vi "積分器(SubVI).vi"(6 "輸入累加ERR回朔":dbl, 7 "I增益":dbl=0.01, 9 "samples (Hz)":dbl, 10 "前一個ERR":dbl, 11 "當下ERR":dbl) -> (1 "輸出累加ERR回朔":dbl, 3 "積分修正量":dbl)   [LabVIEW 2010]
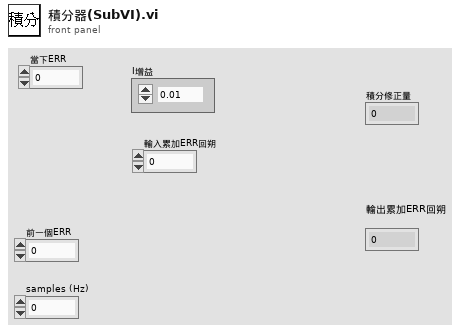
[diagram p1: front panel]
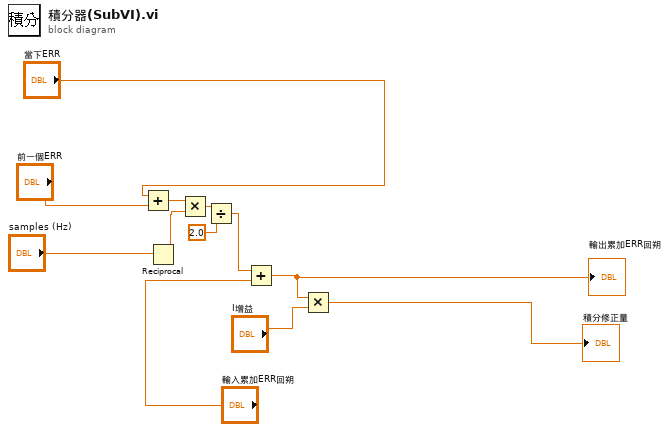
[diagram p0: block diagram]
diagram:
  n1 = Add(x="當下ERR", y="前一個ERR") -> (x+y=w1:dbl)
  n2 = Reciprocal(x="samples (Hz)") -> (1/x=w10:dbl)
  n3 = Multiply(x=w1, y=w10) -> (x*y=w2:dbl)
  n4 = Divide(x=w2, y=2.0) -> (x/y=w5:dbl)
  n5 = Add(x=w5, y="輸入累加ERR回朔") -> (x+y=w7:dbl)
  "輸出累加ERR回朔" <- w7
  n6 = Multiply(x=w7, y="I增益") -> (x*y=→"積分修正量":dbl)
